vi "Catch Nested Value Update.vi"(8 "error in (no error)":errorcluster, 10 "Nested Value Update Msg":refnum<class "Nested Value Update Msg.lvclass">, 11 "tableactor In":refnum<class "tableactor.lvclass">) -> (0 "error out":errorcluster, 3 "tableactor Out":refnum<class "tableactor.lvclass">)   [LabVIEW 2017, in "tableactor.lvlib" / "tableactor.lvclass"]
doc: "<License>\nCopyright © 2017 Composed Systems, LLC | All rights reserved\nwww.composed.io\n\nAuthor: Ethan Stern <ethan.stern@composed.io>\n\nThis software is provided \"AS IS\" WITHOUT WARRANTIES, either express or implied, AND IS FOR EDUCATIONAL PURPOSES ONLY.\n</License>"
uses:
  <userlib>/composed/example/Test/Integration Test/tableactor/tableactor/tableactor.lvclass
  C:/Program Files/National Instruments/LabVIEW 2017/user.lib/composed/mva-viewable/Source/IViewable/IViewable/IViewable.lvclass
  <userlib>/composed/mva-viewable/Source/IViewable/IViewable Messages/Catch Nested Value Change Msg/Nested Value Update Msg.lvclass
  <userlib>/composed/mva-viewable/Source/IViewable/IViewable Messages/Catch Nested Value Change Msg/Nested Value Update Msg.lvclass/Nested Value Update Msg.ctl
  <userlib>/composed/mva-dialogbox/source/DialogBoxViewManager/DialogBoxViewManager/DialogBoxViewManager.lvclass
  <vilib>/Utility/Data Type/NI_Data Type.lvlib
  <userlib>/composed/mva-dialogbox/source/OneButtonDialogBox/OneButtonDialogBox.lvclass
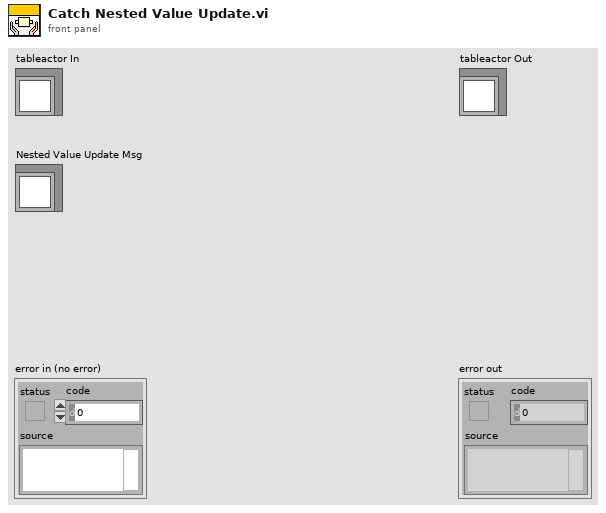
[diagram p1: front panel]
types:
  T1 = typedef "NI_Data Type.lvlib/Data Type.ctl" = enum8{"Invalid Type", "Void", "I8", "I16", "I32", "I64", "U8", "U16", "U32", "U64", "Single Float", "Double Float", "Extended Float", "Single Complex", "Double Complex", "Extended Complex", "Enum U8", "Enum U16", "Enum U32", "Enum U64", "Single Float With Unit", "Double Float With Unit", "Extended Float With Unit", "Single Complex with Unit", "Double Complex with Unit", "Extended Complex with Unit", "Boolean", "String", "Path", "Picture", "Tag", "Array", "Cluster", "Variant", "LV Variant", "Waveform", "Timestamp", "Digital Waveform", "Digital Data", "ExpressData", "Refnum", "External Data", "VI", "Poly VI", "LabVIEW Class Instance", "Fixed Point"}
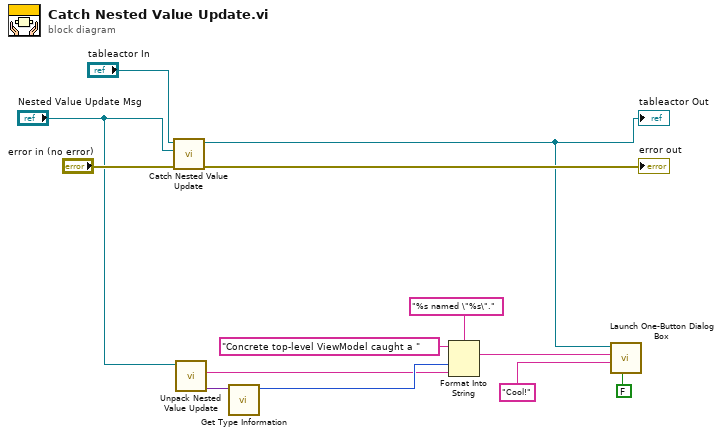
[diagram p0: block diagram]
diagram:
  n1 = call-parent "Catch Nested Value Update.vi"("error in (no error)"="error in (no error)", "Nested Value Update Msg"="Nested Value Update Msg", "IViewable In"="tableactor In") -> ("error out"=→"error out":errorcluster, "IViewable Out"=w1:refnum<class "tableactor.lvclass">)  [unwired: 7 in]
  "tableactor Out" <- w1
  n2 = call <userlib>:"Unpack Nested Value Update.vi"("Nested Value Update Msg"="Nested Value Update Msg") -> ("Value"=w7:variant, "Datum Name"=w6:string)  [unwired: 8 in, 1 out]
  n3 = call <vilib>:"Get Type Information.vi"("Variant"=w7) -> ("Type"=w8:T1)  [unwired: 6 in, 4 out]
  n4 = Format Into String(format string="%s named \"%s\".", initial string="Concrete top-level ViewModel caught a ", w8, w6) -> (resulting string=w5:string)  [unwired: 1 in, 1 out]
  n5 = call <userlib>:"Launch One-Button Dialog Box.vi"("Modal? (T)"=FALSE, "Button Text (OK)"="Cool!", "Message Text"=w5, "Dialog Launcher"=w1) -> ()  [unwired: 7 in, 1 out]
